vi "Write Transmission Data Unit.vi"(8 "error in (no error)":errorcluster, 10 "transmission data unit":refnum<class "Transmission Data Unit.lvclass">, 11 "Modbus instance in":refnum<class "Modbus API.lvclass">) -> (0 "error out":errorcluster, 3 "Modbus instance out":refnum<class "Modbus API.lvclass">)   [LabVIEW 2020, in "SubVIs.lvlib" / "Modbus API.lvclass"]
doc: "This VI is an accessor for the transmission data unit stored in the modbus instance. This accessor can be used as a property node. The transmission data unit is used by the device to determine how to pack and unpack data coming from the physical bus."
uses:
  <vilib>/Modbus/subvis/Modbus API/Modbus API.lvclass
  <vilib>/Modbus/subvis/Transmission Data Unit (ADU)/Transmission Data Unit/Transmission Data Unit.lvclass
  <vilib>/Modbus/subvis/Modbus API/Modbus API.lvclass/Modbus API.ctl
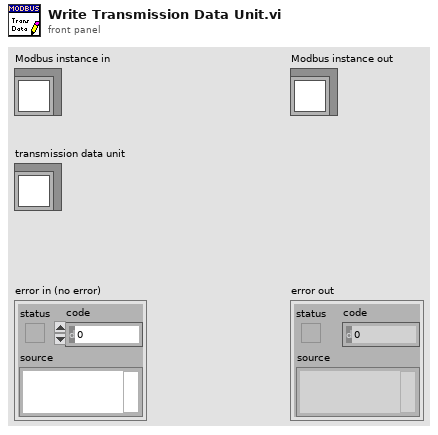
[diagram p1: front panel]
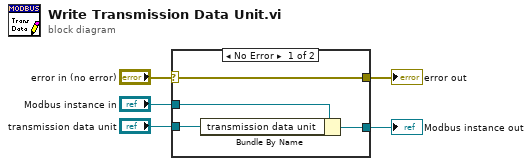
[diagram p0: block diagram]
diagram:
  n1 = case shown="No Error" "error in (no error)" {
    selector: "error in (no error)" -> [w9 w10]
    tunnel: [w9 w10] -> w4
    tunnel: [w7 w11] -> w2
    tunnel: "Modbus instance in" -> [w8 w11]
    tunnel: "transmission data unit" -> [w6 _]
    frame No Error {
      n2 = Bundle By Name(cluster=w8, "transmission data unit"=w6) -> (w7:refnum<class "Modbus API.lvclass">)
    }
    frame Error {
    }
  }
  "error out" <- w4
  "Modbus instance out" <- w2
